vi "delay1min.vi"(1 "error in":errorcluster, 2 "InputData":T1) -> (0 "error out":errorcluster)   [LabVIEW 2010]
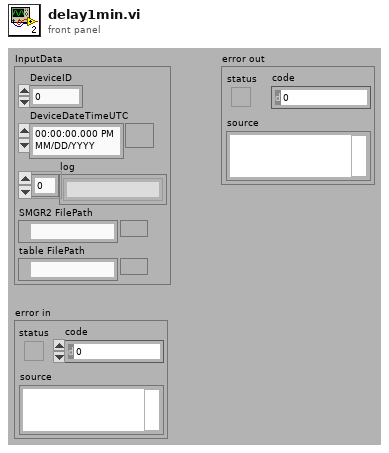
[diagram p1: front panel]
types:
  T1 = cluster{"DeviceID":i32, "DeviceDateTimeUTC":timestamp, "log":string[], "SMGR2 FilePath":path, "table FilePath":path}
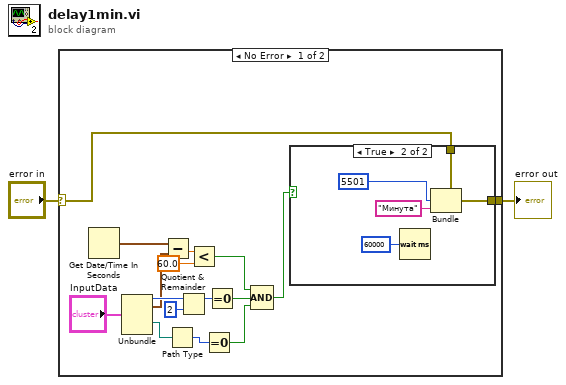
[diagram p0: block diagram]
diagram:
  n1 = case shown="No Error" "error in" {
    selector: "error in" -> [w16 w25]
    tunnel: [w17 w25] -> w2
    frame No Error {
      n2 = Get Date/Time In Seconds() -> (seconds since 1Jan1904=w12:timestamp)
      n3 = Unbundle("InputData") -> ("DeviceID"=w15:i32, "DeviceDateTimeUTC"=w11:timestamp, "SMGR2 FilePath"=w8:path)  [unwired: 2 out]
      n4 = Subtract(x=w12, y=w11) -> (x-y=w10:dbl)
      n5 = Path Type(1:w8) -> (0:w7:i16)
      n6 = Quotient & Remainder(x=w15, y=2) -> (x-y*floor(x/y)=w13:i32)  [unwired: 1 out]
      n7 = Less?(x=w10, y=60.0) -> (x < y?=w4:bool)
      n8 = Equal To 0?(x=w7) -> (x = 0?=w6:bool)
      n9 = Equal To 0?(x=w13) -> (x = 0?=w5:bool)
      n10 = Compound Arithmetic op=AND(w4, w5, w6) -> (w3:bool)
      n11 = case shown="True" w3 {
        tunnel: [w19 w24] -> w17
        tunnel: w16 -> [w19 w23]
        frame False {
        }
        frame True {
          n12 = Wait (ms)(milliseconds to wait=u32 60000) -> ()  [unwired: 1 out]
          n13 = Bundle(cluster=w23, "code"=5501, "source"="Минута") -> (w24:errorcluster)  [unwired: 1 in]
        }
      }
    }
    frame Error {
    }
  }
  "error out" <- w2
